vi "Destroy System Ref.vi"(8 "error in (no error)":errorcluster, 11 "JKI SMO System":refnum<data-value>) -> (0 "error out":errorcluster)   [LabVIEW 2019, in "Registry-SMO.lvclass"]
doc: "JKI State Machine Objects (SMO) 1.3.0.56\nJKI - JKI\nCopyright (c) 2017, JKI"
uses:
  Registry-SMO.lvclass
  Registry-SMO.lvclass/Registry-SMO.ctl
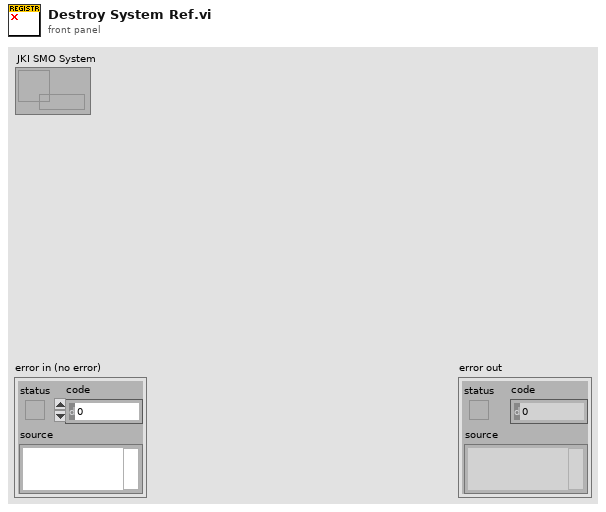
[diagram p1: front panel]
types:
  T1 = typedef "Registry-SMO.lvclass/PublicRegistryEvents--Cluster.ctl" = cluster{"Register Event":refnum<user-event>, "Unregister Event":refnum<user-event>}
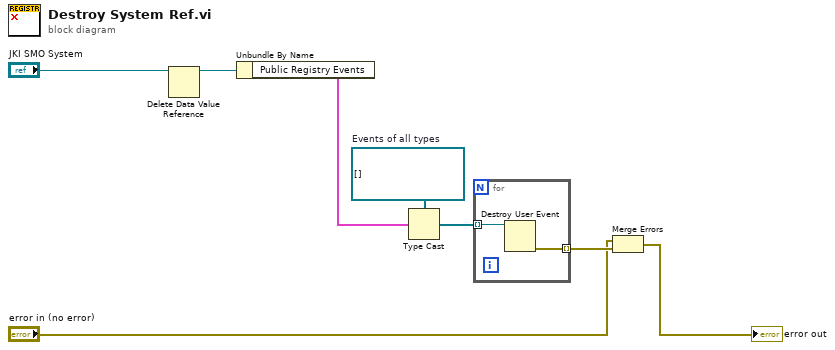
[diagram p0: block diagram]
diagram:
  w6 = refnum<user-event>[] []  # Events of all types
  n1 = Delete Data Value Reference(data value reference="JKI SMO System") -> (data value=w7:refnum<class "Registry-SMO.lvclass">)  [unwired: 1 in, 1 out]
  n2 = Unbundle By Name(w7) -> ("Public Registry Events"=w3:T1)
  n3 = Type Cast(type=w6, x=w3) -> (*(type *) &x=w5:refnum<user-event>[])
  n4 = for {
    tunnel: w5 -> [w10] mode=indexing
    tunnel: [w9] -> w4 mode=indexing
    n5 = Destroy User Event(user event=w10) -> (error out=w9:errorcluster)  [unwired: 1 in]
  }
  n6 = Merge Errors("error in (no error)", w4) -> (→"error out":errorcluster)
